vi "UI Event Handler.vi"() -> ()   [LabVIEW 2017]
panel:
  out "현재 시간":timestamp
  in  "시간 확인":bool
  out "반복":i32
  in  "정지":bool
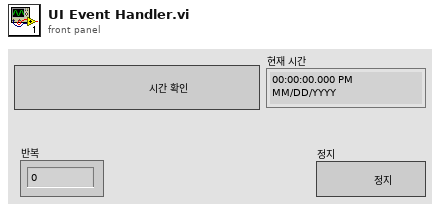
[diagram p1: front panel]
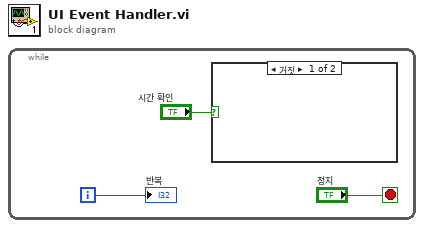
[diagram p0: block diagram]
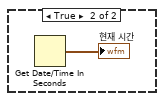
[diagram p2: hidden frame]
diagram:
  n1 = while {
    i -> [w2]
    stop <- "정지" stop-if-true
    n2 = case shown="거짓" "시간 확인" {
      frame False {
      }
      frame True {
        n3 = Get Date/Time In Seconds() -> (seconds since 1Jan1904=→"현재 시간":timestamp)
      }
    }
    "반복" <- w2
  }
